vi "get_config.vi"(4 "error in (no error)":errorcluster, 5 "py interface file":path, 6 "Request data":variant, 7 "Python session in":refnum<k35>) -> (0 "error out":errorcluster, 2 "Response data":variant, 3 "Python session out":refnum<k35>)   [LabVIEW 2022 SP3]
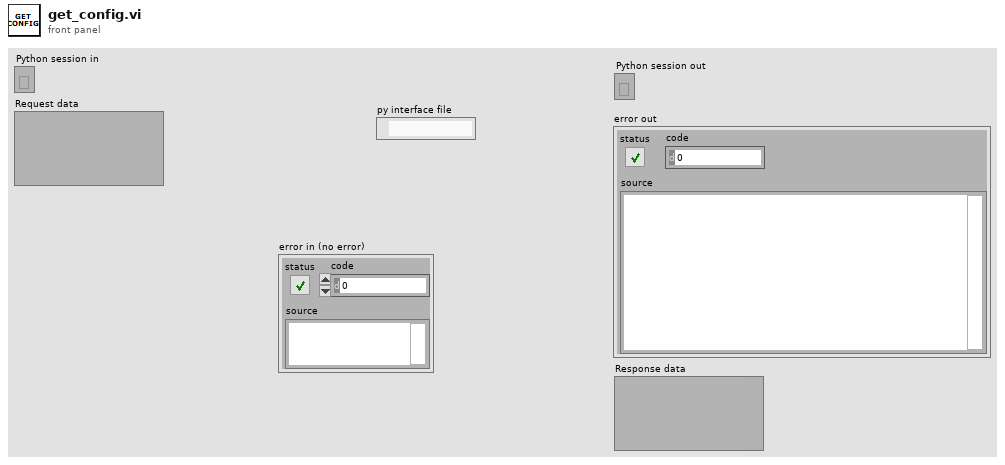
[diagram p1: front panel]
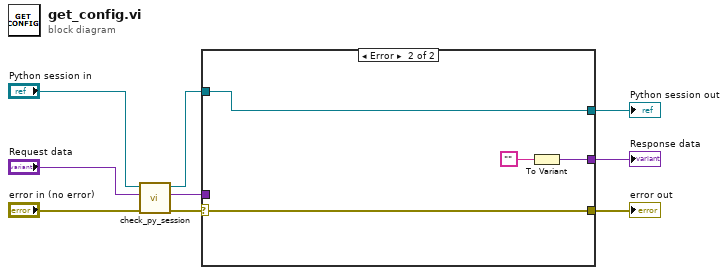
[diagram p0: block diagram]
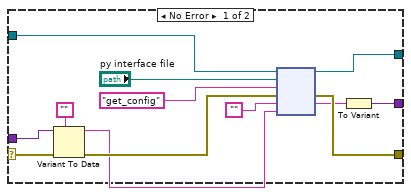
[diagram p2: hidden frame]
diagram:
  n1 = call "check_py_session.vi"("error in"="error in (no error)", "Request data"="Request data", "Python session in"="Python session in") -> ("error out"=w3:errorcluster, "Response data"=w4:variant, "Python session out"=w5:refnum<k35>)  [unwired: 2 in]
  n2 = case shown="Error" w3 {
    selector: w3 -> [w17 w26]
    tunnel: w5 -> [w22 w25]
    tunnel: [w19 w25] -> w9
    tunnel: w4 -> [w18 _]
    tunnel: [w15 w26] -> w2
    tunnel: [w13 w23] -> w1
    frame No Error {
      n3 = Variant To Data(error in=w17, type="", Variant=w18) -> (data=w10:string, error out=w16:errorcluster)
      n4 = node(w22, "py interface file", "get_config" ("function name"), w16, "", w10) -> (w19:refnum<k35>, w15:errorcluster, w14:string)  [unwired: 1 in, 2 out]
      n5 = To Variant(anything=w14) -> (Variant=w13:variant)
    }
    frame Error {
      n6 = To Variant(anything="") -> (Variant=w23:variant)
    }
  }
  "error out" <- w2
  "Python session out" <- w9
  "Response data" <- w1
